vi "Butterfly_PullDown Capacitance.vi"(0 "Semiconductor Module Context":T2, 1 "Capacitance":bool=TRUE, 3 "RFPins":string[](array[string]), 4 "VNAs Measurement Parameters":T1, 5 "error in (no error)":errorcluster, 7 "C_TH_Delta":dbl=2.0, 8 "R Thresholds":dbl[](array[numeric]), 9 "Start_v":dbl=10.0 format="%#_13g", 11 "Stop_v":dbl=41.0 format="%#_13g") -> (14 "Semiconductor Module Context Out":T2, 19 "error out":errorcluster)   [LabVIEW 2013]
uses:
  <vilib>/NI_TestStand_SemiconductorModule/NI_TestStand_Semiconductor_Module.lvlibp/PinMap/General/SemiconductorModuleContext.ctl
  VNA/VNAs Measurement Parameters.ctl
  <instrlib>/niDCPower/nidcpower.llb/niDCPower Wait For Event - Event.ctl
  <vilib>/NI_TestStand_SemiconductorModule/NI_TestStand_Semiconductor_Module.lvlibp/PinMap/DC Power/PinToNIDCPowerSessions.vi
  <vilib>/NI_TestStand_SemiconductorModule/NI_TestStand_Semiconductor_Module.lvlibp/PinMap/General/Publish/PublishDataDoubleFunctionalTest.vi
  <vilib>/NI_TestStand_SemiconductorModule/NI_TestStand_Semiconductor_Module.lvlibp/PinMap/General/Publish/PublishDataDouble2D.vi
  <vilib>/NI_TestStand_SemiconductorModule/NI_TestStand_Semiconductor_Module.lvlibp
  VNA/Pin Map API/VNA Custom Instrument.lvlib
panel:
  out "C_Free":dbl[](array[numeric])
  out "VRLs":dbl[][](array[numeric]) format="%#_3g"
  out "VPIs":dbl[][](array[numeric]) format="%#_3g"
  out "appended array":dbl[][](array[numeric]) format="%#_3g"
  out "S3 steps":dbl[](array[numeric]) format="%#_3g"
  out "S2 steps":dbl[](array[numeric]) format="%#_3g"
  out "S1 steps":dbl[](array[numeric]) format="%#_3g"
  out "S0 steps":dbl[](array[numeric]) format="%#_3g"
  out "BF values":dbl[](array[numeric])
  out "VRLs":dbl[](array[numeric])
  out "VPIs":dbl[](array[numeric])
  out "Multisite Cap Data":dbl[][][](array[numeric])
  out "Full Array":dbl[][][](array[numeric])
  out "BF Names":string[](array[string])
  in  "current level":dbl=0.01 format="%_6p"
  out "R Array":dbl[](array[numeric])
  out "BFSamples":i32
  in  "Step_v":dbl=1.0
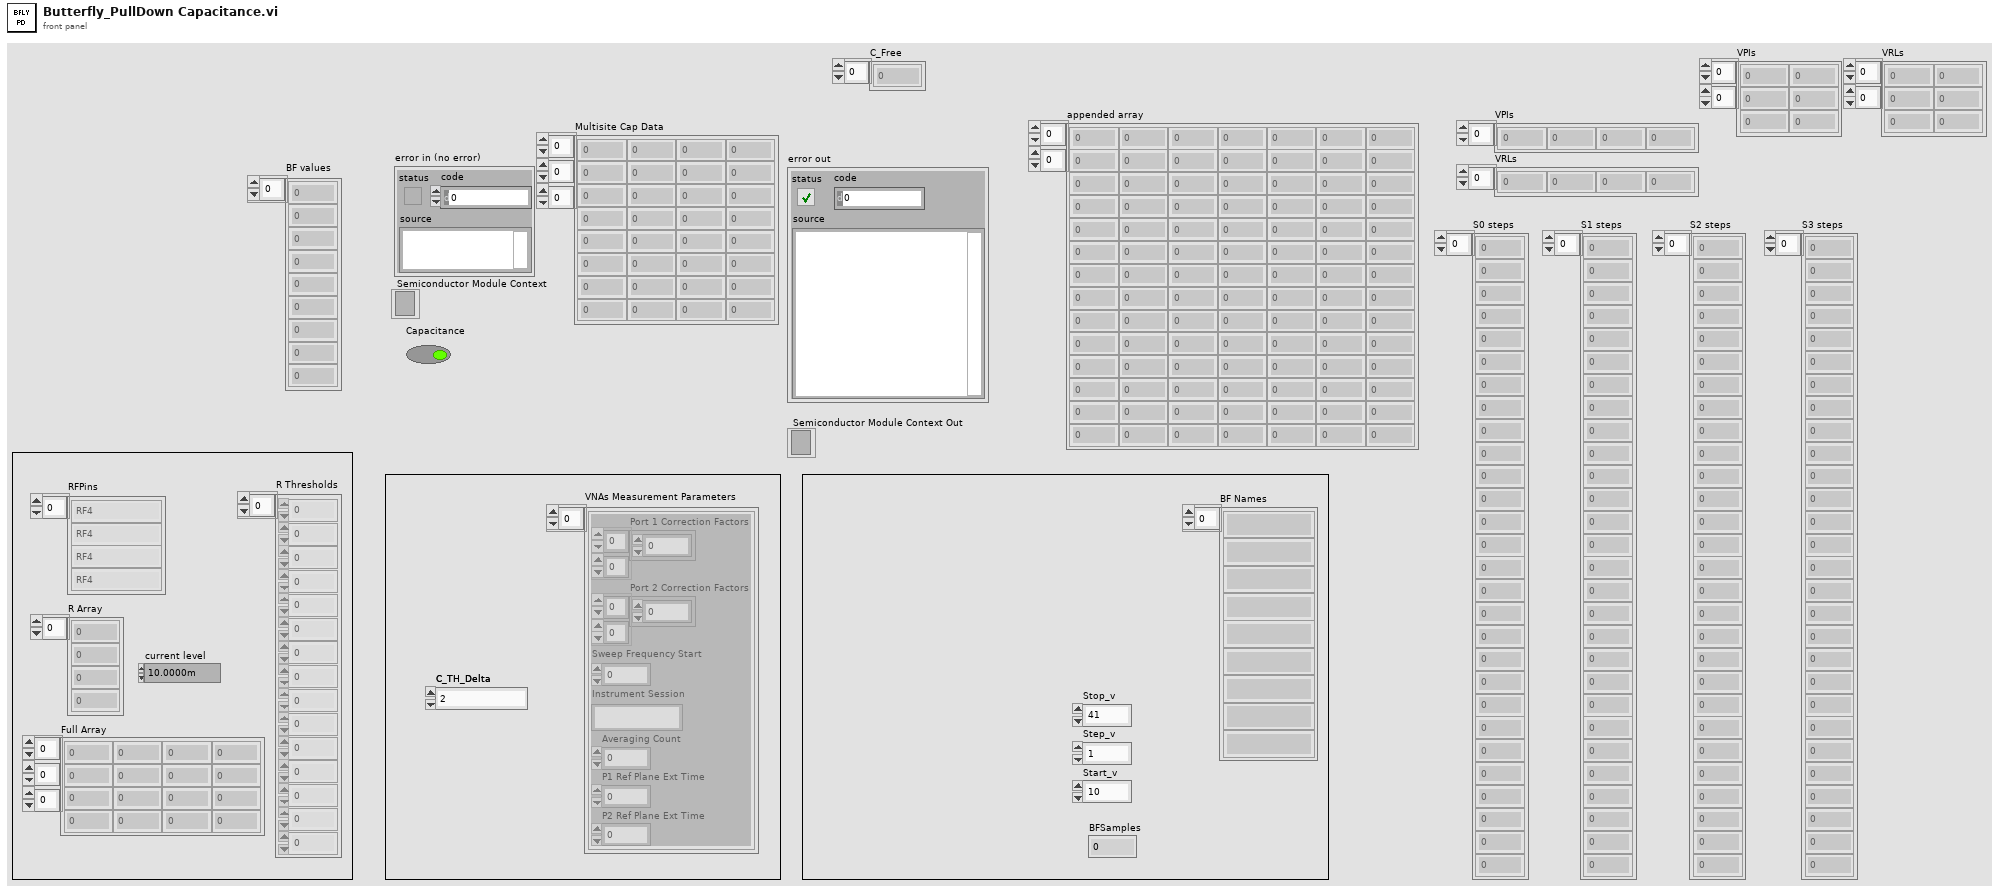
[diagram p1: front panel]
types:
  T1 = typedef "VNAs Measurement Parameters.ctl" = cluster{"Port 1 Correction Factors":cdb[][], "Port 2 Correction Factors":cdb[][], "Sweep Frequency Start":dbl, "Instrument Session":string, "Averaging Count":i32, "P1 Ref Plane Ext Time":dbl, "P2 Ref Plane Ext Time":dbl}[]
  T2 = typedef "NI_TestStand_Semiconductor_Module.lvlibp/SemiconductorModuleContext.ctl" = refnum<k7>
  T3 = typedef "niDCPower Wait For Event - Event.ctl" = i32
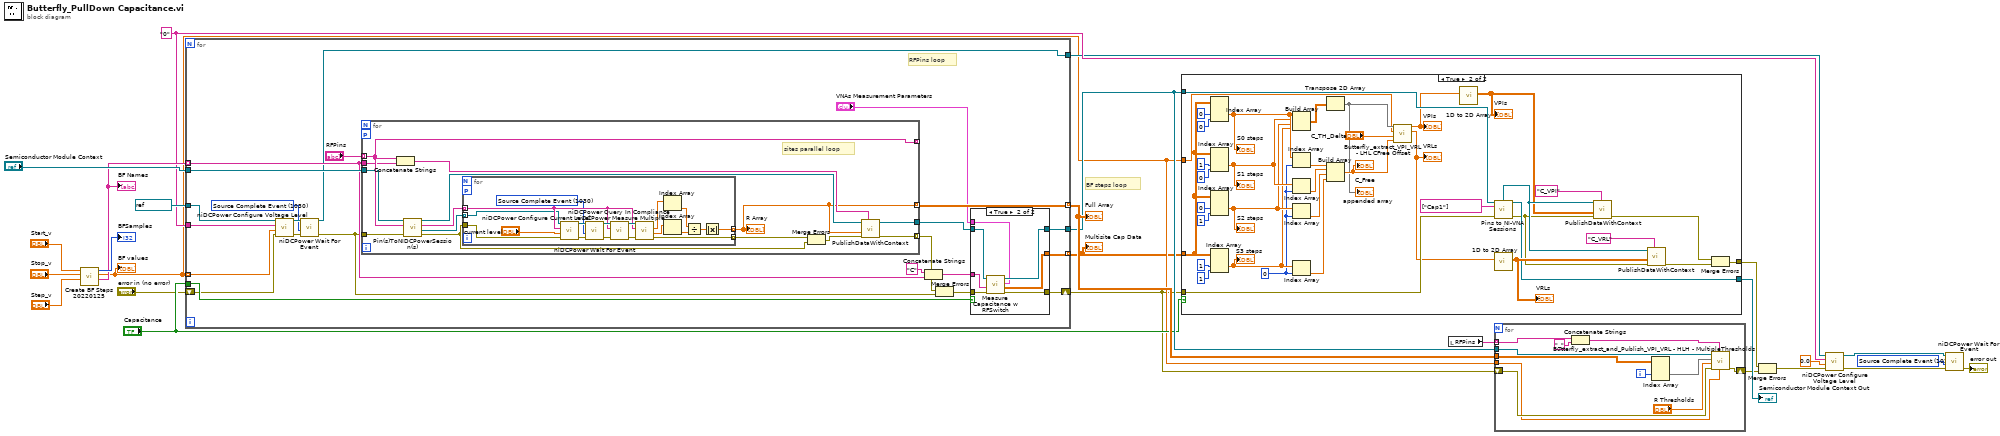
[diagram p0: block diagram]
diagram:
  w7 = T3 1030 items=["Source Complete Event"=1030, "Measure Complete Event"=1031, "Sequence Iteration Complete Event"=1032, "Sequence Engine Done Event"=1033, "Pulse Complete Event"=1051, "Ready For Pulse Trigger Event"=1052] ("event")
  w12 = "0" ("channel name")
  # "BF steps loop"
  n1 = call "Create BF Steps 20220125.vi"("Step_v"="Step_v", "Stop_v"="Stop_v", "Start_v"="Start_v") -> ("BF Names"=w16:string[], "BF values"=w6:dbl[], "BFSamples"=→"BFSamples":i32)  [unwired: 6 in]
  "BF Names" <- w16
  "BF values" <- w6
  n2 = for {
    shift-right: [w27] -> w4
    shift-left: "error in (no error)" -> [w33]
    tunnel: [w49] -> w25 mode=indexing
    tunnel: "Semiconductor Module Context" -> [w47]
    tunnel: [w45] -> w22
    tunnel: [w41] -> w5 mode=indexing
    tunnel: "Capacitance" -> [w38]
    tunnel: w16 -> [w37] mode=indexing
    tunnel: w6 -> [w31] mode=indexing
    tunnel: w12 -> [w30]
    tunnel: refnum<k15> "4139_1" ("instrument handle") -> [w29]
    tunnel: [w28] -> w11
    w35 = T3 1030 items=["Source Complete Event"=1030, "Measure Complete Event"=1031, "Sequence Iteration Complete Event"=1032, "Sequence Engine Done Event"=1033, "Pulse Complete Event"=1051, "Ready For Pulse Trigger Event"=1052] ("event")
    # "RFPins loop"
    n3 = call <instrlib>:"niDCPower Configure Voltage Level.vi"("error in (no error)"=w33, "voltage level"=w31, "channel name"=w30, "instrument handle"=w29) -> ("error out"=w34:errorcluster, "instrument handle out"=w36:refnum<k15>)  [unwired: 6 in]
    n4 = call <instrlib>:"niDCPower Wait For Event.vi"("error in (no error)"=w34, "event"=w35, "instrument handle"=w36) -> ("error out"=w32:errorcluster, "instrument handle out"=w28:refnum<k15>)  [unwired: 7 in]
    n5 = for {
      tunnel: [w68] -> w46
      tunnel: "RFPins" -> [w63] mode=indexing
      tunnel: [w64] -> w49 mode=indexing
      tunnel: [w63] -> _ mode=indexing
      tunnel: w47 -> [w61]
      workers-P: _ -> [_]
      tunnel: [w66] -> w40 mode=indexing
      tunnel: w32 -> [w60]
      tunnel: w37 -> [w59]
      # "sites parallel loop"
      n6 = Concatenate Strings(w63, w59) -> (w65:string)
      n7 = call-poly <vilib>:"Pin(s)ToNIDCPowerSession(s).vi"("error in (no error)"=w60, "Pin"=w63, "Semiconductor Module Context"=w61) -> ("error out"=w70:errorcluster, "Instrument Sessions"=w71:refnum<k15>[], "Channel Lists"=w72:string[], "Semiconductor Module Context Out"=w69:T2)  [unwired: 4 in, 1 out]
      n8 = for {
        tunnel: w72 -> [w77] mode=indexing
        tunnel: w71 -> [w73] mode=indexing
        tunnel: w70 -> [w74]
        tunnel: [w78] -> w64 mode=indexing
        workers-P: _ -> [_]
        tunnel: [w75] -> w62 mode=indexing
        w76 = T3 1030 items=["Source Complete Event"=1030, "Measure Complete Event"=1031, "Sequence Iteration Complete Event"=1032, "Sequence Engine Done Event"=1033, "Pulse Complete Event"=1051, "Ready For Pulse Trigger Event"=1052] ("event")
        n9 = call <instrlib>:"niDCPower Configure Current Level.vi"("error in (no error)"=w74, "current level"="current level", "channel name"=w77, "instrument handle"=w73) -> ("error out"=w86:errorcluster, "instrument handle out"=w85:refnum<k15>)  [unwired: 6 in]
        n10 = call <instrlib>:"niDCPower Wait For Event.vi"("error in (no error)"=w86, "event"=w76, "instrument handle"=w85) -> ("error out"=w90:errorcluster, "instrument handle out"=w89:refnum<k15>)  [unwired: 7 in]
        n11 = call <instrlib>:"niDCPower Query In Compliance.vi"("error in (no error)"=w90, "channel name"=w77, "instrument handle"=w89) -> ("error out"=w87:errorcluster, "instrument handle out"=w88:refnum<k15>)  [unwired: 6 in, 1 out]
        n12 = call <instrlib>:"niDCPower Measure Multiple.vi"("error in (no error)"=w87, "channel name"=w77, "instrument handle"=w88) -> ("error out"=w75:errorcluster, "current measurements"=w79:dbl[], "voltage measurements"=w80:dbl[])  [unwired: 5 in, 1 out]
        n13 = Index Array(array=w80) -> (element=w82:dbl)  [unwired: 1 in]
        n14 = Index Array(array=w79) -> (element=w81:dbl)  [unwired: 1 in]
        n15 = Divide(x=w82, y=w81) -> (x/y=w83:dbl)
        n16 = Absolute Value(x=w83) -> (abs(x)=w78:dbl)
      }
      "R Array" <- w64
      n17 = Merge Errors(w62, w70) -> (w67:errorcluster)
      n18 = call-poly <vilib>:"PublishDataWithContext.vi"("Published Data Id"=w65, "error in (no error)"=w67, "Data In"=w64, "Semiconductor Module Context"=w69) -> ("error out"=w66:errorcluster, "Semiconductor Module Context Out"=w68:T2)  [unwired: 6 in]
    }
    n19 = Concatenate Strings("C" ("string"), w37) -> (w43:string)
    n20 = Merge Errors(w40, w32) -> (w39:errorcluster)
    n21 = case shown="True" w38 {
      tunnel: w46 -> [w51 w58]
      tunnel: [w51 w57] -> w45
      tunnel: [w50 w56] -> w27
      tunnel: w43 -> [_ w55]
      tunnel: "VNAs Measurement Parameters" -> [_ w54]
      tunnel: [_ w53] -> w41
      tunnel: w39 -> [w50 w52]
      frame False {
      }
      frame True {
        n22 = call "Measure Capacitance w RFSwitch.vi"("VNAs Measurement Parameters"=w54, "error in (no error)"=w52, "Measurement Id"=w55, "Semiconductor Module Context"=w58) -> ("error out"=w56:errorcluster, "Multisite Cap Data"=w53:dbl[][], "Semiconductor Module Context Out"=w57:T2)  [unwired: 5 in]
      }
    }
  }
  "Full Array" <- w25
  "Multisite Cap Data" <- w5
  n23 = case shown="True" "Capacitance" {
    tunnel: [w91 w111] -> w23
    tunnel: [w92 w129] -> w3
    tunnel: w22 -> [w91 w128]
    tunnel: w4 -> [w92 w124]
    tunnel: w6 -> [_ w96]
    tunnel: w5 -> [_ w115]
    frame False {
    }
    frame True {
      w104 = 0 ("index")
      n24 = Index Array(array=w115, index (dim 1)=0 ("disabled index (row)"), index (dim 2)=0 ("disabled index (col)")) -> (element=w108:dbl[])  [unwired: 1 in]
      "S0 steps" <- w108
      n25 = Index Array(array=w115, index (dim 1)=1 ("index (row)"), index (dim 2)=0 ("index (col)")) -> (element=w107:dbl[])  [unwired: 1 in]
      "S1 steps" <- w107
      n26 = Index Array(array=w115, index (dim 1)=0 ("index (row)"), index (dim 2)=1 ("index (col)")) -> (element=w106:dbl[])  [unwired: 1 in]
      "S2 steps" <- w106
      n27 = Index Array(array=w115, index (dim 1)=1 ("index (row)"), index (dim 2)=1 ("index (col)")) -> (element=w105:dbl[])  [unwired: 1 in]
      "S3 steps" <- w105
      n28 = Build Array(w108, w107, w106, w105) -> (w99:dbl[][])
      n29 = Index Array(array=w108, index=w104) -> (element=w103:dbl)
      n30 = Index Array(array=w107, index=w104) -> (element=w102:dbl)
      n31 = Index Array(array=w106, index=w104) -> (element=w101:dbl)
      n32 = Index Array(array=w105, index=w104) -> (element=w100:dbl)
      n33 = Transpose 2D Array(2D array=w99) -> (transposed array=w97:dbl[][])
      "appended array" <- w97
      n34 = Build Array(w103, w102, w101, w100) -> (w98:dbl[])
      "C_Free" <- w98
      n35 = call "Butterfly_extract_VPI_VRL - LHL CFree Offset.vi"("C_Free"=w98, "Delta"="C_TH_Delta", "Voltage Array"=w96, "Result Array In"=w97) -> ("VRLs"=w93:dbl[], "VPIs"=w94:dbl[])  [unwired: 6 in]
      "VPIs" <- w94
      "VRLs" <- w93
      n36 = call "1D to 2D Array.vi"("1D Array"=w94) -> ("2D Array"=w113:dbl[][])  [unwired: 10 in]
      "VPIs" <- w113
      n37 = call "Pins to NI-VNA Sessions.vi"("Semiconductor Module Context"=w128, "Pins"=string[] ["Cap1"] ("Capacitance Pins"), "error in (no error)"=w124) -> ("Pin Query Context"=w114:refnum<class "MultiplePinMultipleSessionQueryContext.lvclass">, "Semiconductor Module Context Out"=w111:T2, "error out"=w109:errorcluster)  [unwired: 8 in, 2 out]
      n38 = call "1D to 2D Array.vi"("1D Array"=w93) -> ("2D Array"=w127:dbl[][])  [unwired: 10 in]
      "VRLs" <- w127
      n39 = call-poly <vilib>:"PublishDataWithContext.vi"("Published Data Id"="C_VPI", "error in (no error)"=w109, "Data In"=w113, "Pin Query Context"=w114) -> ("error out"=w110:errorcluster)  [unwired: 6 in, 1 out]
      n40 = call-poly <vilib>:"PublishDataWithContext.vi"("Published Data Id"="C_VRL", "error in (no error)"=w109, "Data In"=w127, "Pin Query Context"=w114) -> ("error out"=w130:errorcluster)  [unwired: 6 in, 1 out]
      n41 = Merge Errors(w110, w130) -> (w129:errorcluster)
    }
  }
  "Semiconductor Module Context Out" <- w23
  n42 = local read "RFPins"() -> (w26:string[])
  n43 = for {
    tunnel: w26 -> [w135] mode=indexing
    tunnel: w25 -> [w140]
    shift-right: [w136] -> w2
    shift-left: w4 -> [w137]
    tunnel: w22 -> [w132]
    tunnel: w6 -> [w131]
    i -> [w141]
    n44 = Concatenate Strings(w135, "_" ("string")) -> (w133:string)
    n45 = Index Array(array=w140, index (dim 1)=w141) -> (element=w138:dbl[][])  [unwired: 2 in]
    n46 = call "Butterfly_extract_and_Publish_VPI_VRL - HLH - MultipleThresholds.vi"("Voltages Array"=w131, "ID Prefix"=w133, "error in (no error)"=w137, "Thresholds"="R Thresholds", "Result Array In"=w138, "Semiconductor Module Context"=w132) -> ("error out"=w136:errorcluster)  [unwired: 5 in]
  }
  n47 = Merge Errors(w3, w2) -> (w1:errorcluster)
  n48 = call <instrlib>:"niDCPower Configure Voltage Level.vi"("error in (no error)"=w1, "voltage level"=0.0, "channel name"=w12, "instrument handle"=w11) -> ("error out"=w10:errorcluster, "instrument handle out"=w8:refnum<k15>)  [unwired: 6 in]
  n49 = call <instrlib>:"niDCPower Wait For Event.vi"("error in (no error)"=w10, "event"=w7, "instrument handle"=w8) -> ("error out"=→"error out":errorcluster)  [unwired: 7 in, 1 out]
